vi "-8024 Receive queue was read too late--error.vi"(8 "error in":errorcluster, 11 "Argument":string) -> (0 "error out":errorcluster, 2 "Error Code":i32)   [LabVIEW 2018, in "PCANBasic.lvlib"]
uses:
  PCANBasic.lvlib
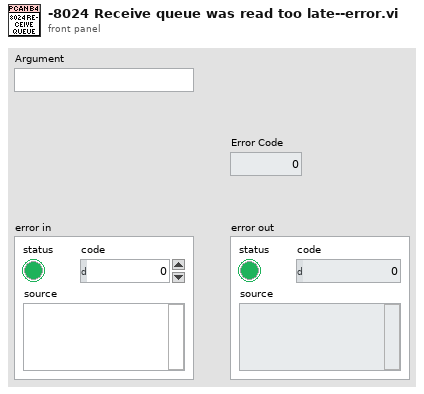
[diagram p1: front panel]
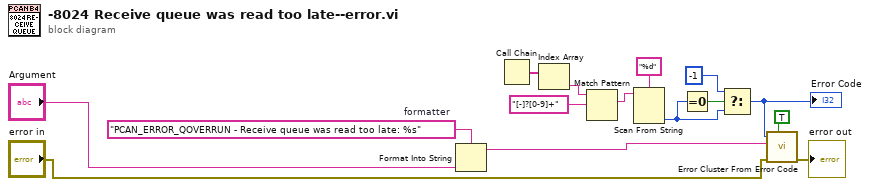
[diagram p0: block diagram]
diagram:
  w12 = "PCAN_ERROR_QOVERRUN - Receive queue was read too late: %s"  # formatter
  n1 = Format Into String(format string=w12, "Argument") -> (resulting string=w13:string)  [unwired: 2 in, 1 out]
  n2 = Call Chain() -> (call chain=w3:string[])
  n3 = Index Array(array=w3) -> (element=w8:string)  [unwired: 1 in]
  n4 = Match Pattern(string=w8, regular expression="[-]?[0-9]+") -> (match substring=w9:string)  [unwired: 1 in, 3 out]
  n5 = Scan From String(format string="%d", input string=w9) -> (output 1=w5:i32)  [unwired: 3 in, 3 out]
  n6 = Equal To 0?(x=w5) -> (x = 0?=w6:bool)
  n7 = Select(t=-1, s=w6, f=w5) -> (s? t:f=w2:i32)
  "Error Code" <- w2
  n8 = call <vilib>:"Error Cluster From Error Code.vi"("show call chain? (False)"=TRUE, "error in (no error)"="error in", "error message (\"\")"=w13, "error code (0)"=w2) -> ("error out"=→"error out":errorcluster)  [unwired: 5 in]
